vi "Initialize Process Queues Map.vi"(8 "Error In":errorcluster, 10 "Processes Queues":refnum<queue>[](array[refnum]), 11 "Central Message Handler In":refnum<class "Central Message Handler.lvclass">) -> (0 "Error Out":errorcluster, 3 "Central Message Handler Out":refnum<class "Central Message Handler.lvclass">)   [LabVIEW 2019, in "Central Message Handler.lvclass"]
uses:
  Central Message Handler.lvclass
  Process/Public/Controls/Process Message.ctl
  Accessors/Processes Queues Map/Set Processes Queues Map.vi
  Process/Process.lvclass
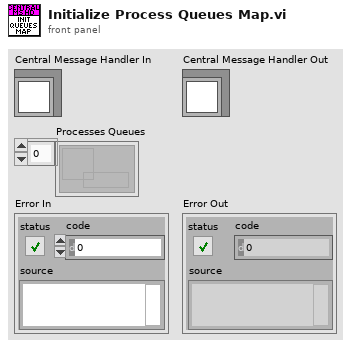
[diagram p1: front panel]
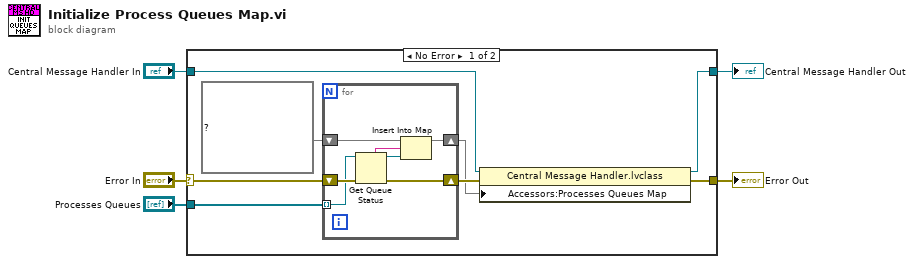
[diagram p0: block diagram]
diagram:
  n1 = case shown="No Error" "Error In" {
    selector: "Error In" -> [w12 w22]
    tunnel: [w8 w22] -> w4
    tunnel: "Central Message Handler In" -> [w13 w21]
    tunnel: [w9 w21] -> w2
    tunnel: "Processes Queues" -> [w11 _]
    frame No Error {
      n2 = for {
        tunnel: w11 -> [w19] mode=indexing
        shift-right: [w16] -> w6
        shift-left: map{string, refnum<queue>} {} ("Processes Queues Map") -> [w17]
        shift-right: [w15] -> w10
        shift-left: w12 -> [w20]
        n3 = Get Queue Status(queue=w19, error in (no error)=w20) -> (queue out=w14:refnum<queue>, queue name=w18:string, error out=w15:errorcluster)  [unwired: 1 in, 5 out]
        n4 = Insert Into Map(map in=w17, key=w18, value=w14) -> (map out=w16:map{string, refnum<queue>})  [unwired: 2 out]
      }
      n5 = property class="Central Message Handler.lvclass"(reference=w13, error in=w10, "Accessors:Processes Queues Map"=w6) -> (reference out=w9:refnum<class "Central Message Handler.lvclass">, error out=w8:errorcluster)
    }
    frame Error {
    }
  }
  "Central Message Handler Out" <- w2
  "Error Out" <- w4
